vi "INICIA_SERIAL_AQUISICAO.vi"() -> ()   [LabVIEW 2018]
uses:
  <vilib>/Instr/_visa.llb/VISA Configure Serial Port (Instr).vi
  Global_Telescopio.vi
panel:
  out "AQUISICAO  RESOURCE":refnum<visa-resource-name>
  in  "flow control (0:none)":u16(ring) items=["None", "XON/XOFF", "RTS/CTS", "XON/XOFF & RTS/CTS", "DTR/DSR", "XON/XOFF & DTR/DSR"]
  in  "stop bits (10: 1 bit)":u16(ring)=10 items=["1.0"=10, "1.5"=15, "2.0"=20]
  in  "parity (0:none)":enum16{"None", "Odd", "Even", "Mark", "Space"}(ring)
  in  "baud rate (2400)":u32=2400
  in  "VISA resource name":refnum<visa-resource-name>="COM65"
  # "COM 65 NECESSÁRIA"
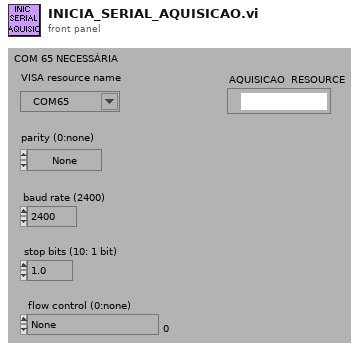
[diagram p1: front panel]
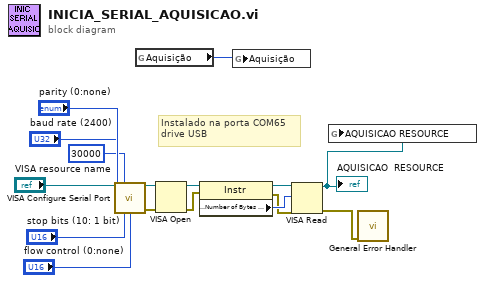
[diagram p0: block diagram]
diagram:
  # "Instalado na porta COM65\ndrive USB"
  n1 = call-poly "VISA Configure Serial Port"("VISA resource name"="VISA resource name", "timeout (10sec)"=u32 30000, "baud rate (9600)"="baud rate (2400)", "parity (0:none)"="parity (0:none)", "stop bits (10: 1 bit)"="stop bits (10: 1 bit)", "flow control (0:none)"="flow control (0:none)") -> ("VISA resource name out"=w10:refnum<visa-resource-name>, "error out"=w11:errorcluster)  [unwired: 8 in]
  n2 = global read "Global_Telescopio.vi" "Aquisição"() -> (w1:i32)
  n3 = VISA Open(error in (no error)=w11, VISA resource name=w10) -> (VISA resource name=w15:refnum<visa-resource-name>, error out=w16:errorcluster)  [unwired: 3 in]
  n4 = property class="Instr"(reference=w15, error in=w16) -> (reference out=w12:refnum<visa-resource-name>, error out=w13:errorcluster, "Serial Settings:Number of Bytes at Serial Port"=w14:u32)
  n5 = global write "Global_Telescopio.vi" "Aquisição"(w1) -> ()
  n6 = VISA Read(VISA resource name=w12, byte count=w14, error in (no error)=w13) -> (VISA resource name out=w2:refnum<visa-resource-name>, error out=w3:errorcluster)  [unwired: 2 out]
  "AQUISICAO  RESOURCE" <- w2
  n7 = global write "Global_Telescopio.vi" "AQUISICAO RESOURCE"(w2) -> ()
  n8 = call <vilib>:"General Error Handler.vi"("error in (no error)"=w3) -> ()  [unwired: 10 in, 5 out]
